vi "GetTagByProperties.vi"(10 "properties":T1[](array[typedef]), 11 "tags":T2[](array[typedef])) -> (1 "found":bool, 2 "tag":T2, 3 "tags out":T2[](array[typedef]))   [LabVIEW 2017, in "DeviceModelHelpers.lvlib"]
doc: "Returns a tag based on the specified properties."
uses:
  <vilib>/addons/InsightCM/Utilities/DeviceModelHelpers/DeviceModelHelpers.lvlib
  <vilib>/addons/InsightCM/MessageBus/Base/controls/Tag.ctl
  <vilib>/addons/InsightCM/MessageBus/Base/controls/KeyValuePair.ctl
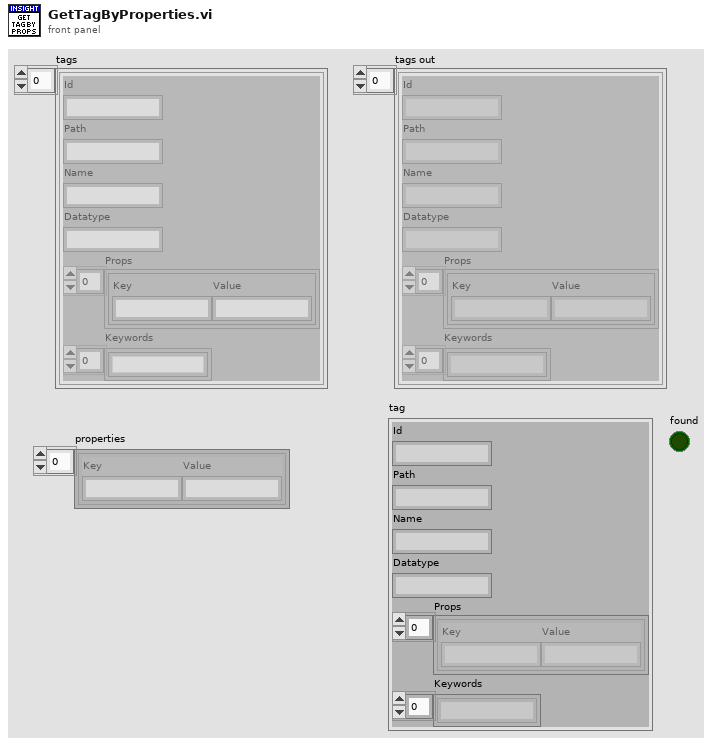
[diagram p1: front panel]
types:
  T1 = typedef "KeyValuePair.ctl" = cluster{"Key":string, "Value":string}
  T2 = typedef "Tag.ctl" = cluster{"Id":string, "Path":string, "Name":string, "Datatype":string, "Props":T1[], "Keywords":string[]}
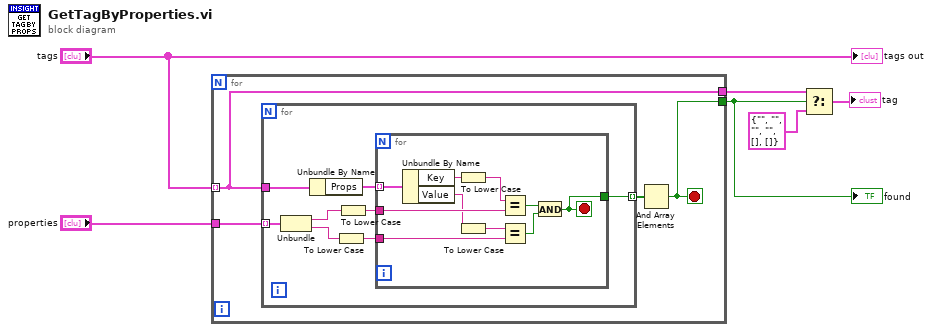
[diagram p0: block diagram]
diagram:
  n1 = for {
    tunnel: "tags" -> [w10] mode=indexing
    tunnel: [w7] -> w4
    tunnel: [w10] -> w3
    tunnel: "properties" -> [w9]
    stop <- w7 stop-if-true
    n2 = for {
      tunnel: w10 -> [w17]
      tunnel: w9 -> [w14] mode=indexing
      tunnel: [w11] -> w8 mode=indexing
      n3 = Unbundle(w14) -> ("Key"=w13:string, "Value"=w12:string)
      n4 = Unbundle By Name(w17) -> ("Props"=w18:T1[])
      n5 = To Lower Case(string=w12) -> (all lower case string=w16:string)
      n6 = To Lower Case(string=w13) -> (all lower case string=w15:string)
      n7 = for {
        tunnel: w15 -> [w28]
        tunnel: [w21] -> w11
        tunnel: w18 -> [w27] mode=indexing
        tunnel: w16 -> [w23]
        stop <- w21 stop-if-true
        n8 = Unbundle By Name(w27) -> ("Key"=w25:string, "Value"=w24:string)
        n9 = To Lower Case(string=w25) -> (all lower case string=w20:string)
        n10 = To Lower Case(string=w24) -> (all lower case string=w19:string)
        n11 = Equal?(x=w20, y=w28) -> (x = y?=w26:bool)
        n12 = Equal?(x=w19, y=w23) -> (x = y?=w22:bool)
        n13 = And(x=w26, y=w22) -> (x .and. y?=w21:bool)
      }
    }
    n14 = And Array Elements(Boolean array=w8) -> (logical AND=w7:bool)
  }
  "found" <- w4
  n15 = Select(t=w3, s=w4, f=T2 {"Id"="", "Path"="", "Name"="", "Datatype"="", "Props"=[], "Keywords"=[]}) -> (s? t:f=→"tag":T2)
  "tags out" <- "tags"
